vi "Binary Saving Module.vi"(5 "action":string="Save", 8 "error in":errorcluster, 10 "file path (use dialog)":path, 11 "data in":sgl[](array[numeric])) -> (0 "error out":errorcluster)   [LabVIEW 2018]
uses:
  Controls/Queue Manager Actions.ctl
  Controls/QueueNames.ctl
  Controls/MessagePacket.ctl
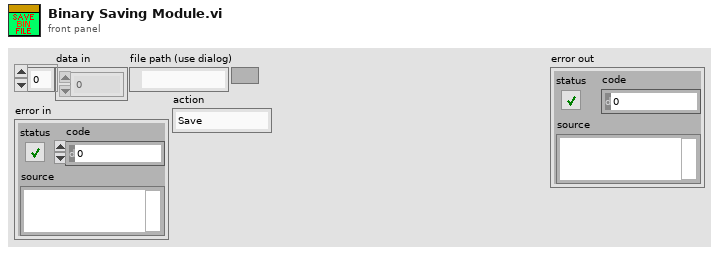
[diagram p1: front panel]
types:
  T1 = typedef "MessagePacket.ctl" = cluster{"Message":string, "Parameter":variant}
  T2 = typedef "QueueNames.ctl" = enum16{"Main GUI", "Main Scan Processor", "Main Processing", "Main Saving", "Main Display", "Main Table Stage GUI", "Main Table Stage Proc.", "Scan Engine", "Vibratome GUI", "Vibratome Processor", "Slice Engine"}
  T3 = typedef "Queue Manager Actions.ctl" = enum16{"Init", "Enqueue", "Enqueue All", "Preview Queue", "Dequeue", "Get Status", "Flush Queue", "Flush All Queues", "Release All Queues", "Release Queue", "Enqueue at Opposite End"}
  T4 = enum16{"big-endian, network order", "native, host order", "little-endian"}
  T5 = enum16{"open", "replace", "create", "open or create", "replace or create", "replace or create with confirmation"}
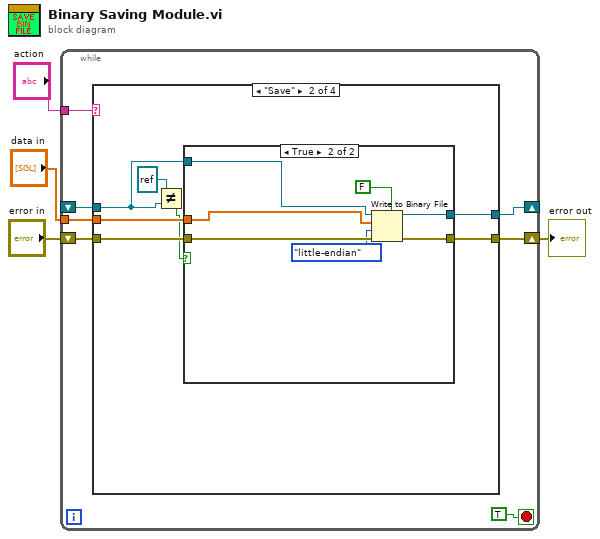
[diagram p0: block diagram]
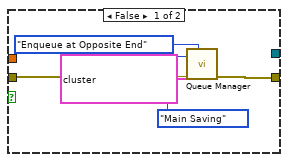
[diagram p3: hidden frame]
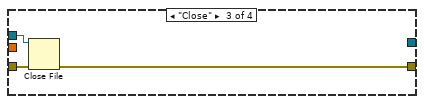
[diagram p4: hidden frame]
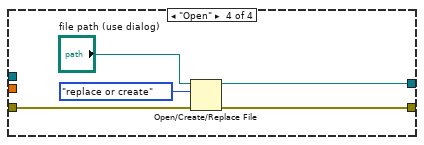
[diagram p5: hidden frame]
diagram:
  n1 = while {
    tunnel: "action" -> [w10]
    tunnel: "data in" -> [w9]
    shift-right: [w7] -> w2
    shift-left: "error in" -> [w8]
    shift-right: [w6] -> _
    shift-left: _ -> [w5]
    stop <- TRUE stop-if-true
    n2 = case shown="\"Save\"" w10 {
      tunnel: w9 -> [_ w17 _ _]
      tunnel: w8 -> [w13 w18 w35 w39]
      tunnel: [w13 w20 w34 w37] -> w7
      tunnel: [w12 w19 _ w40] -> w6
      tunnel: w5 -> [w12 w14 w33 _]
      frame "False", Default {
      }
      frame "Save" {
        n3 = Not Equal?(x=refnum<file> refnum ("refnum out"), y=w14) -> (x != y?=w15:bool)
        n4 = case shown="True" w15 {
          tunnel: [w21 w32] -> w20
          tunnel: [_ w31] -> w19
          tunnel: w18 -> [w22 w30]
          tunnel: w17 -> [_ w27]
          tunnel: w14 -> [_ w26]
          frame False {
            n5 = call "Queue Manager.vi"("Queue Name"=QueueNames."Main Saving", "Action"=Queue_Manager_Actions."Enqueue at Opposite End", "Error In"=w22, "Message Packet Array"=T1[] [{"Message"="Save", "Parameter"=variant}, {"Message"="Open", "Parameter"=variant}]) -> ("Error Out"=w21:errorcluster)  [unwired: 3 in, 4 out]
          }
          frame True {
            n6 = Write to Binary File(file (use dialog)=w26, data=w27, error in=w30, 5:FALSE ("prepend array or string size? (T)"), 9:T4."little-endian" ("byte order (0:big-endian, network order)")) -> (refnum out=w31:refnum<file>, error out=w32:errorcluster)  [unwired: 1 in, 1 out]
          }
        }
      }
      frame "Close" {
        n7 = Close File(refnum=w33, error in=w35) -> (error out=w34:errorcluster)  [unwired: 1 out]
      }
      frame "Open" {
        n8 = Open/Create/Replace File(file path (use dialog)="file path (use dialog)", error in=w39, operation (0:open)=T5."replace or create") -> (refnum out=w40:refnum<file>, error out=w37:errorcluster)  [unwired: 3 in, 1 out]
      }
    }
  }
  "error out" <- w2
